vi "handle message.vi"(8 "error in":errorcluster, 10 "message":refnum<class "communicator message.lvclass">, 11 "queue manager in":refnum<class "queue manager.lvclass">) -> (0 "error out":errorcluster, 1 "stop":bool, 3 "queue manager out":refnum<class "queue manager.lvclass">)   [LabVIEW 2015, in "queue manager.lvclass"]
uses:
  queue manager.lvclass
  message/communicator message.lvclass
  message/communicator message.lvclass/communicator message.ctl
  new communicator message.ctl
  communicator/communicator.lvclass
  queue manager.lvclass/queue manager.ctl
  communicator/communicator.lvclass/communicator.ctl
  communicator manager/communicator manager.lvlib
  communicator queue/identifying queue.lvclass
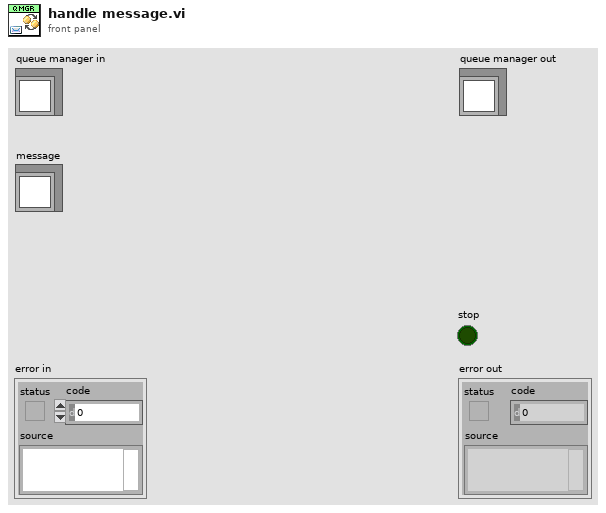
[diagram p1: front panel]
types:
  T1 = typedef "queue manager.lvclass/new communicator message.ctl" = cluster{"ID":string, "comm":refnum<class "communicator.lvclass">}
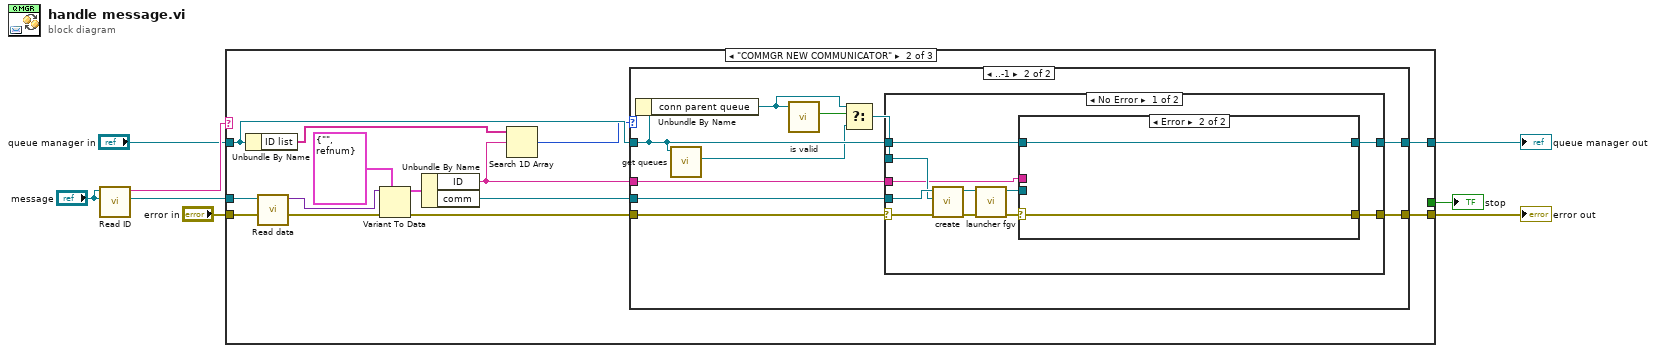
[diagram p0: block diagram]
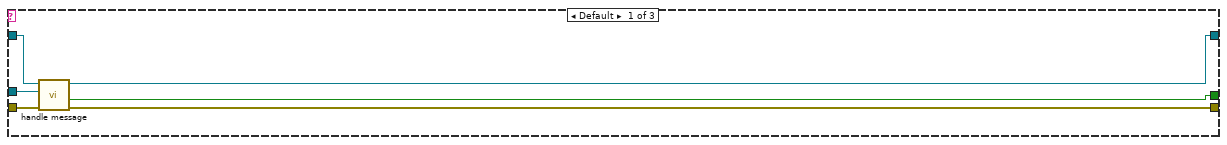
[diagram p2: hidden frame]
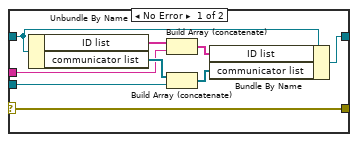
[diagram p4: hidden frame]
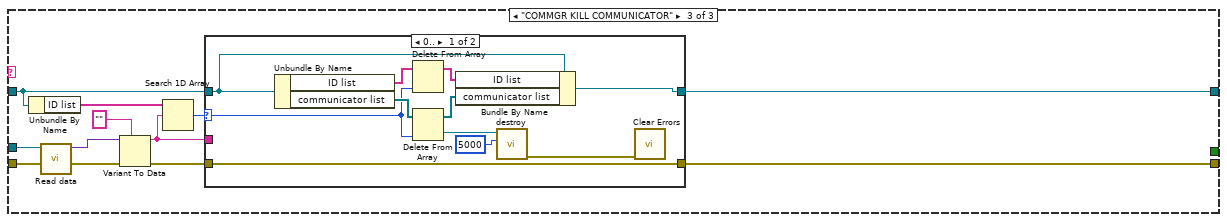
[diagram p6: hidden frame]
diagram:
  n1 = call "Read ID.vi"("communicator message in"="message") -> ("ID"=w7:string)  [unwired: 10 in]
  n2 = case shown="\"COMMGR NEW COMMUNICATOR\"" w7 {
    tunnel: "error in" -> [w13 w26 w73]
    tunnel: [w12 w19 w69] -> w3
    tunnel: "queue manager in" -> [w11 w16 w66]
    tunnel: [w10 w18 w68] -> w5
    tunnel: "message" -> [w8 w25 w72]
    tunnel: [w9 _ _] -> w4
    frame Default {
      n3 = call-parent "handle message.vi"("error in"=w13, "message"=w8, "communicator in"=w11) -> ("error out"=w12:errorcluster, "stop"=w9:bool, "communicator out"=w10:refnum<class "queue manager.lvclass">)  [unwired: 6 in]
    }
    frame "COMMGR NEW COMMUNICATOR" {
      n4 = Unbundle By Name(w16) -> ("ID list"=w17:string[])
      n5 = call "Read data.vi"("communicator message in"=w25) -> ("data"=w24:variant)  [unwired: 10 in]
      n6 = Variant To Data(error in=w26, type=T1 {"ID"="", "comm"=refnum} ("new comm message"), Variant=w24) -> (data=w21:T1, error out=w20:errorcluster)
      n7 = Unbundle By Name(w21) -> ("ID"=w15:string, "comm"=w22:refnum<class "communicator.lvclass">)
      n8 = Search 1D Array(1D array=w17, element=w15) -> (index of element=w14:i32)  [unwired: 1 in]
      n9 = case shown="..-1" w14 {
        tunnel: w22 -> [_ w38]
        tunnel: w20 -> [w28 w37]
        tunnel: [w28 w36] -> w19
        tunnel: [w27 w35] -> w18
        tunnel: w16 -> [w27 w33]
        tunnel: w15 -> [_ w34]
        frame 0.. {
        }
        frame ..-1 {
          n10 = Unbundle By Name(w33) -> ("conn parent queue"=w31:refnum<class "identifying queue.lvclass">)
          n11 = call "get queues.vi"("communicator in"=w33) -> ("to this"=w30:refnum<class "identifying queue.lvclass">)  [unwired: 9 in, 1 out]
          n12 = call "is valid.vi"("identifying queue in"=w31) -> ("valid?"=w32:bool)  [unwired: 9 in, 1 out]
          n13 = Select(t=w31, s=w32, f=w30) -> (s? t:f=w29:refnum<class "identifying queue.lvclass">)
          n14 = case shown="No Error" w37 {
            selector: w37 -> [w45 w62]
            tunnel: w38 -> [w49 _]
            tunnel: w29 -> [w48 _]
            tunnel: [w41 w62] -> w36
            tunnel: [w43 w61] -> w35
            tunnel: w33 -> [w44 w61]
            tunnel: w34 -> [w40 _]
            frame No Error {
              n15 = call "create.vi"("error in"=w45, "parent"=w48, "uninitialized communicator"=w49) -> ("error out"=w47:errorcluster, "communicator out"=w46:refnum<class "communicator.lvclass">)  [unwired: 7 in]
              n16 = call "launcher fgv.vi"("error in"=w47, "communicator in"=w46) -> ("error out"=w42:errorcluster, "initialized communicator"=w39:refnum<class "communicator.lvclass">)  [unwired: 8 in]
              n17 = case shown="Error" w42 {
                selector: w42 -> [w52 w60]
                tunnel: w44 -> [w58 w59]
                tunnel: [w57 w59] -> w43
                tunnel: [w52 w60] -> w41
                tunnel: w40 -> [w50 _]
                tunnel: w39 -> [w51 _]
                frame No Error {
                  n18 = Unbundle By Name(w58) -> ("ID list"=w56:string[], "communicator list"=w55:refnum<class "communicator.lvclass">[])
                  n19 = Build Array (concatenate)(w56, w50) -> (w53:string[])
                  n20 = Build Array (concatenate)(w55, w51) -> (w54:refnum<class "communicator.lvclass">[])
                  n21 = Bundle By Name(cluster=w58, "ID list"=w53, "communicator list"=w54) -> (w57:refnum<class "queue manager.lvclass">)
                }
                frame Error {
                }
              }
            }
            frame Error {
            }
          }
        }
      }
    }
    frame "COMMGR KILL COMMUNICATOR" {
      n22 = Unbundle By Name(w66) -> ("ID list"=w67:string[])
      n23 = call "Read data.vi"("communicator message in"=w72) -> ("data"=w71:variant)  [unwired: 10 in]
      n24 = Variant To Data(error in=w73, type="", Variant=w71) -> (data=w63:string, error out=w70:errorcluster)
      n25 = Search 1D Array(1D array=w67, element=w63) -> (index of element=w65:i32)  [unwired: 1 in]
      n26 = case shown="0.." w65 {
        selector: w65 -> [w77 _]
        tunnel: w70 -> [w82 w86]
        tunnel: [w82 w86] -> w69
        tunnel: [w84 w85] -> w68
        tunnel: w66 -> [w83 w85]
        tunnel: w63 -> [_ _]
        frame 0.. {
          n27 = Unbundle By Name(w83) -> ("ID list"=w79:string[], "communicator list"=w81:refnum<class "communicator.lvclass">[])
          n28 = Delete From Array(array=w79, index=w77) -> (array with subset deleted=w78:string[])  [unwired: 1 in, 1 out]
          n29 = Delete From Array(array=w81, index=w77) -> (deleted portion=w76:refnum<class "communicator.lvclass">, array with subset deleted=w80:refnum<class "communicator.lvclass">[])  [unwired: 1 in]
          n30 = Bundle By Name(cluster=w83, "ID list"=w78, "communicator list"=w80) -> (w84:refnum<class "queue manager.lvclass">)
          n31 = call-dynamic "destroy.vi"("timeout in ms (-1)"=5000, "communicator in"=w76) -> ("error out"=w75:errorcluster)  [unwired: 9 in]
          n32 = call <vilib>:"Clear Errors.vi"("error in (no error)"=w75) -> ()  [unwired: 5 in, 2 out]
        }
        frame ..-1 {
        }
      }
    }
  }
  "error out" <- w3
  "queue manager out" <- w5
  "stop" <- w4
